vi "FGEN Init.vi"(8 "error in (no error)":errorcluster, 10 "Resource Name":refnum<k15>, 11 "Function Generator in":refnum<class "Function Generator.lvclass">) -> (0 "error out":errorcluster, 3 "Function Generator out":refnum<class "Function Generator.lvclass">)   [LabVIEW 2023, in "HardwareAbstractionLayer_LVOOP.lvlib" / "Function Generator.lvclass"]
uses:
  Function Generator.lvclass
  Function Generator.lvclass/Function Generator.ctl
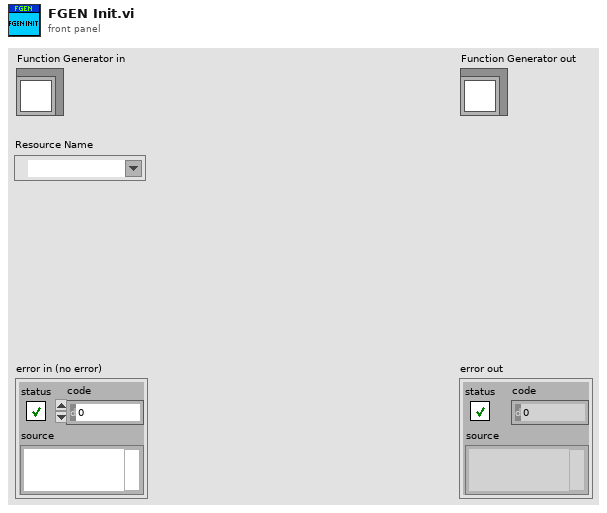
[diagram p1: front panel]
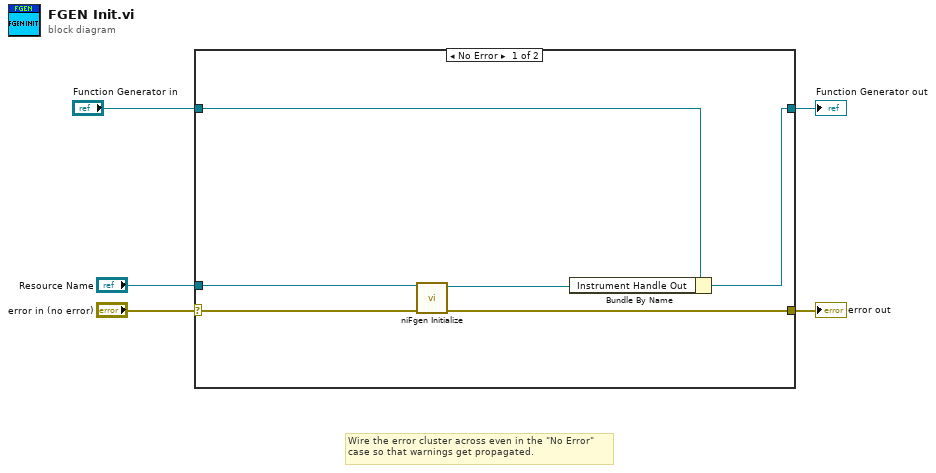
[diagram p0: block diagram]
diagram:
  # "Wire the error cluster across even in the \"No Error\"\ncase so that warnings get propagated."
  n1 = case shown="No Error" "error in (no error)" {
    selector: "error in (no error)" -> [w9 w13]
    tunnel: [w8 w13] -> w4
    tunnel: [w10 w12] -> w2
    tunnel: "Function Generator in" -> [w11 w12]
    tunnel: "Resource Name" -> [w7 _]
    frame No Error {
      n2 = call <instrlib>:"niFgen Initialize.vi"("error in (no error)"=w9, "Resource Name"=w7) -> ("error out"=w8:errorcluster, "Instrument Handle Out"=w6:refnum<k15>)  [unwired: 8 in]
      n3 = Bundle By Name(cluster=w11, "Instrument Handle Out"=w6) -> (w10:refnum<class "Function Generator.lvclass">)
    }
    frame Error {
    }
  }
  "error out" <- w4
  "Function Generator out" <- w2
